vi "Write Port settings.vi"(8 "error in (no error)":errorcluster, 10 "Port settings":T1, 11 "Modbus in":refnum<class "Modbus.lvclass">) -> (0 "error out":errorcluster, 3 "Modbus out":refnum<class "Modbus.lvclass">)   [LabVIEW 2020, in "Modbus.lvlib" / "Modbus.lvclass"]
uses:
  Modbus.lvclass
  Port Settings.ctl
  Modbus.lvclass/Modbus.ctl
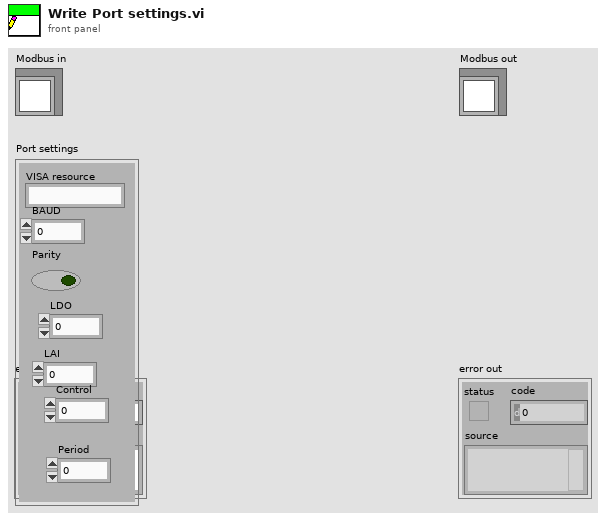
[diagram p1: front panel]
types:
  T1 = typedef "Port Settings.ctl" = cluster{"VISA resource":string, "BAUD":u16, "Parity":bool, "LDO":u16, "LAI":u16, "Control":u16, "Period":u16}
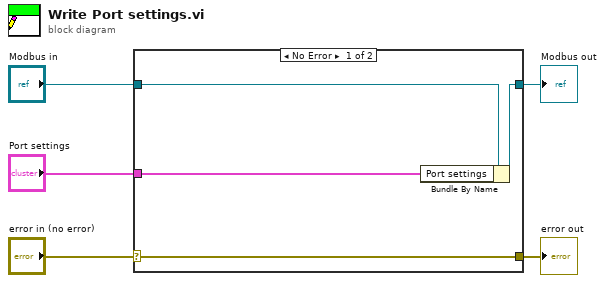
[diagram p0: block diagram]
diagram:
  n1 = case shown="No Error" "error in (no error)" {
    selector: "error in (no error)" -> [w9 w10]
    tunnel: [w9 w10] -> w4
    tunnel: [w7 w11] -> w2
    tunnel: "Modbus in" -> [w8 w11]
    tunnel: "Port settings" -> [w6 _]
    frame No Error {
      n2 = Bundle By Name(cluster=w8, "Port settings"=w6) -> (w7:refnum<class "Modbus.lvclass">)
    }
    frame Error {
    }
  }
  "error out" <- w4
  "Modbus out" <- w2
